vi "Set Controls.vi"(8 "error in (no error)":errorcluster, 10 "Pump Controls":T2 {"Mass Flow SP [kg/h]" min=0.0 max=64.255}, 11 "input cluster":T1={"Session_Control"="Sess_Control", "Session_Params"="Sess_Params", "Session_Actuals"="Sess_Actuals", "Session_Acknowledge"="Sess_Ack", "Session_H2_Sensor"="H2_Sensor_Session", "Session_DILICO_MeasurementRequest"="Session_DILICO_MeasurementRequest", "Session_DILICO_Voltages"="Session_DILICO_Voltages"}) -> (0 "error out":errorcluster, 3 "output cluster":T1={"Session_Control"="Session_Control", "Session_Params"="Session_Params", "Session_Actuals"="Session_Actuals", "Session_Acknowledge"="Session_Acknowledge", "Session_H2_Sensor"="H2_Sensor_Session", "Session_DILICO_MeasurementRequest"="Session_DILICO_MeasurementRequest", "Session_DILICO_Voltages"="Session_DILICO_Voltages"})   [LabVIEW 2025, in "phlair-busch-can-bus.lvlib"]
uses:
  phlair-busch-can-bus.lvlib
  CAN Frame Sessions.ctl
  <vilib>/xnet/xnet.llb/XNET Write (Signal Single-point).vi
  <resource>/objmgr/xnet.rc
  PumpControls.ctl
panel:
  out "Array 2":u32[](array[numeric])
  out "Array":dbl[](array[numeric])
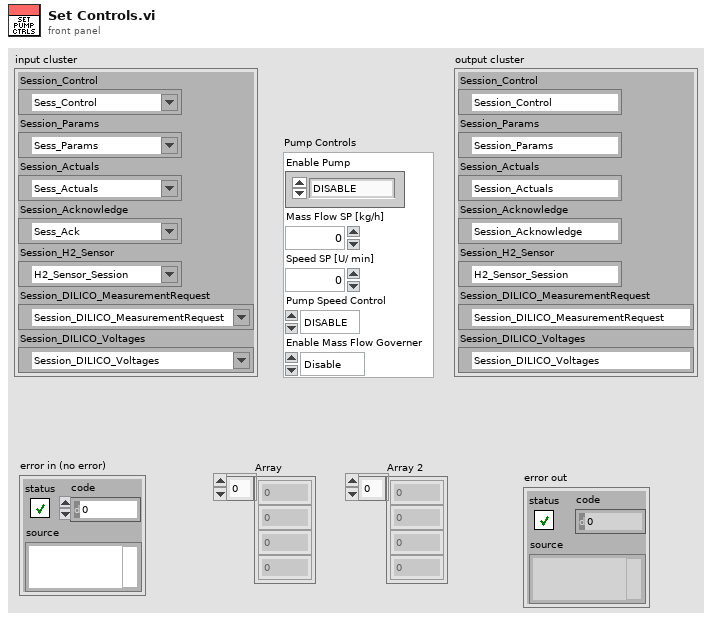
[diagram p1: front panel]
types:
  T1 = typedef "phlair-busch-can-bus.lvlib/CAN Frame Sessions.ctl" = cluster{"Session_Control":refnum<k21>, "Session_Params":refnum<k21>, "Session_Actuals":refnum<k21>, "Session_Acknowledge":refnum<k21>, "Session_H2_Sensor":refnum<k21>, "Session_DILICO_MeasurementRequest":refnum<k21>, "Session_DILICO_Voltages":refnum<k21>}
  T2 = typedef "phlair-busch-can-bus.lvlib/PumpControls.ctl" = cluster{"Enable Pump":enum16{"DISABLE", "ENABLE"}, "Mass Flow SP [kg/h]":dbl, "Speed SP [U/ min]":u16, "Pump Speed Control":enum16{"DISABLE", "ENABLE"}, "Enable Mass Flow Governer":enum8{"Disable", "Enable", "", "NA"}}
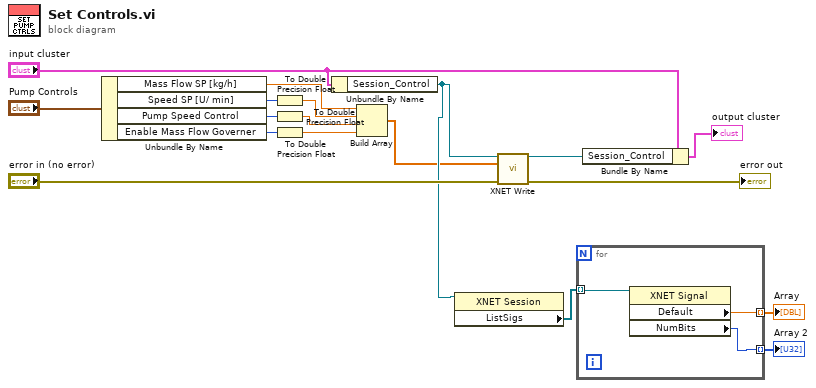
[diagram p0: block diagram]
diagram:
  n1 = Unbundle By Name("Pump Controls") -> ("Mass Flow SP [kg/h]"=w15:dbl, "Speed SP [U/ min]"=w14:u16, "Pump Speed Control"=w13:enum16{"DISABLE", "ENABLE"}, "Enable Mass Flow Governer"=w12:enum8{"Disable", "Enable", "", "NA"})
  n2 = To Double Precision Float(number=w14) -> (double precision float=w11:dbl)
  n3 = To Double Precision Float(number=w13) -> (double precision float=w10:dbl)
  n4 = To Double Precision Float(number=w12) -> (double precision float=w9:dbl)
  n5 = Unbundle By Name("input cluster") -> ("Session_Control"=w5:refnum<k21>)
  n6 = Build Array(w15, w11, w10, w9) -> (w1:dbl[])
  n7 = property class="XNET Session"(reference=w5) -> ("ListSigs"=w4:refnum<k21>[])  [unwired: 1 in, 2 out]
  n8 = call-poly <vilib>:"XNET Write.vi"("session in"=w5, "data"=w1, "error in (no error)"="error in (no error)") -> ("session out"=w6:refnum<k21>, "error out"=→"error out":errorcluster)  [unwired: 11 in]
  n9 = for {
    tunnel: w4 -> [w21] mode=indexing
    tunnel: [w20] -> w3 mode=indexing
    tunnel: [w19] -> w2 mode=indexing
    n10 = property class="XNET Signal"(reference=w21) -> ("Default"=w20:dbl, "NumBits"=w19:u32)  [unwired: 1 in, 2 out]
  }
  "Array" <- w3
  "Array 2" <- w2
  n11 = Bundle By Name(cluster="input cluster", "Session_Control"=w6) -> (→"output cluster":T1)
